vi "Start Server.vi"(8 "error in":errorcluster, 11 "gRPC server in":refnum<class "Servicer.lvclass">) -> (0 "error out":errorcluster, 2 "Listening Port":i32, 3 "gRPC server out":refnum<class "Servicer.lvclass">)   [LabVIEW 2019, in "gRPC-servicer.lvlib" / "Servicer.lvclass"]
uses:
  Servicer.lvclass
  Servicer.lvclass/Servicer.ctl
  gRPC lv Support/grpc-lvsupport.lvlib
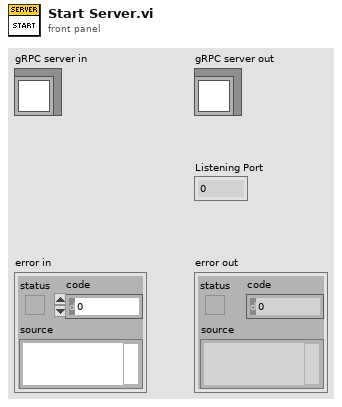
[diagram p1: front panel]
types:
  T1 = typedef "grpc-lvsupport.lvlib/grpcId.ctl" = u64
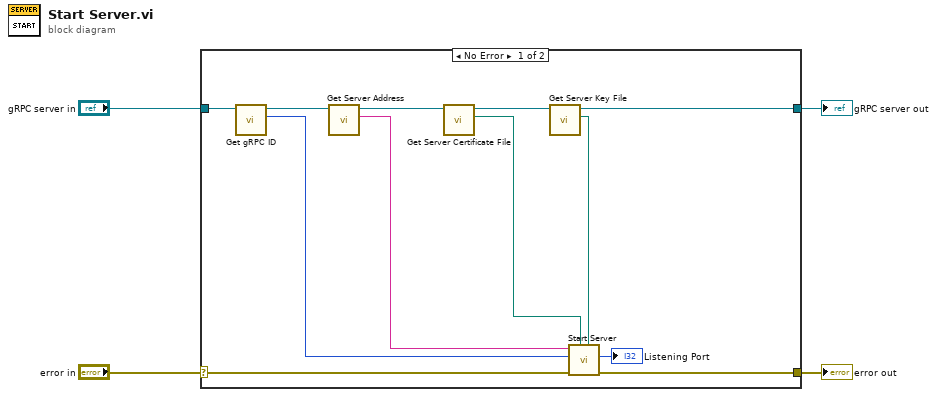
[diagram p0: block diagram]
diagram:
  n1 = case shown="No Error" "error in" {
    selector: "error in" -> [w16 w18]
    tunnel: [w15 w18] -> w3
    tunnel: [w6 w17] -> w1
    tunnel: "gRPC server in" -> [w13 w17]
    frame No Error {
      n2 = call "Get gRPC ID.vi"("gRPC server in"=w13) -> ("gRPC ID"=w11:T1, "gRPC server out"=w12:refnum<class "Servicer.lvclass">)  [unwired: 9 in]
      n3 = call "Get Server Address.vi"("gRPC server in"=w12) -> ("Server Address"=w14:string, "gRPC server out"=w10:refnum<class "Servicer.lvclass">)  [unwired: 9 in]
      n4 = call "Get Server Certificate File.vi"("gRPC server in"=w10) -> ("Server Certificate File (.crt)"=w9:path, "gRPC server out"=w8:refnum<class "Servicer.lvclass">)  [unwired: 9 in]
      n5 = call "Get Server Key File.vi"("gRPC server in"=w8) -> ("Server Key File (.key)"=w7:path, "gRPC server out"=w6:refnum<class "Servicer.lvclass">)  [unwired: 9 in]
      n6 = call "Start Server.vi"("Server Key File (.key)"=w7, "Server Certificate File (.crt)"=w9, "error in"=w16, "gRPCid server in"=w11, "Server Address"=w14) -> ("error out"=w15:errorcluster, "Listening Port"=→"Listening Port":i32)  [unwired: 4 in, 1 out]
    }
    frame Error {
    }
  }
  "error out" <- w3
  "gRPC server out" <- w1
